vi "Close Server.vi"(8 "error in (no error)":errorcluster, 11 "Base Server in":refnum<class "Server.lvclass">) -> (0 "error out":errorcluster, 3 "Base Server out":refnum<class "Server.lvclass">)   [LabVIEW 2024, in "Ramses Framework.lvlib" / "Server.lvclass"]
uses:
  Server.lvclass
  Server.lvclass/Server.ctl
  Write Server Running.vi
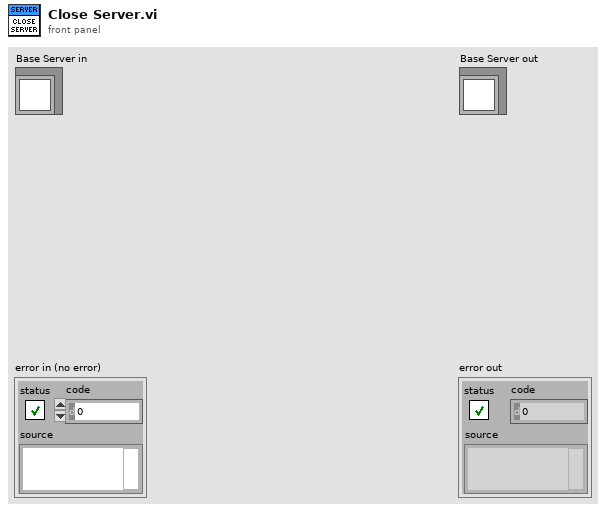
[diagram p1: front panel]
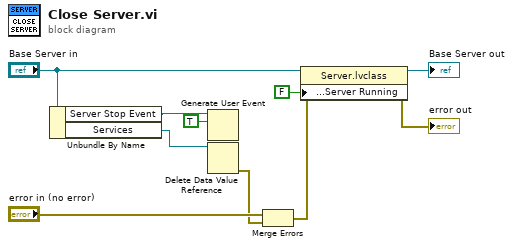
[diagram p0: block diagram]
diagram:
  n1 = Unbundle By Name("Base Server in") -> ("Server Stop Event"=w8:refnum<user-event>, "Services"=w6:refnum<data-value>)
  n2 = Generate User Event(user event=w8, event data cluster=TRUE ("event data")) -> ()  [unwired: 2 in, 2 out]
  n3 = Delete Data Value Reference(data value reference=w6) -> (error out=w5:errorcluster)  [unwired: 1 in, 1 out]
  n4 = Merge Errors("error in (no error)", w5) -> (w2:errorcluster)
  n5 = property class="Server.lvclass"(reference="Base Server in", error in=w2, "Public API:Accessors:Server Running"=FALSE ("Server Running")) -> (reference out=→"Base Server out":refnum<class "Server.lvclass">, error out=→"error out":errorcluster)
